vi "HW_Server.vi"(8 "Error In":errorcluster) -> (0 "Error Out":errorcluster)   [LabVIEW 2011]
doc: "This VI will handle communication with Main VI and HW."
uses:
  SubVIs/Controls/TransparencyEffectOperations.ctl
  SubVIs/Controls/Global Stop - Operations.ctl
  SubVIs/Controls/INIT- READ - WRITE.ctl
panel:
  # "HW SERVER"
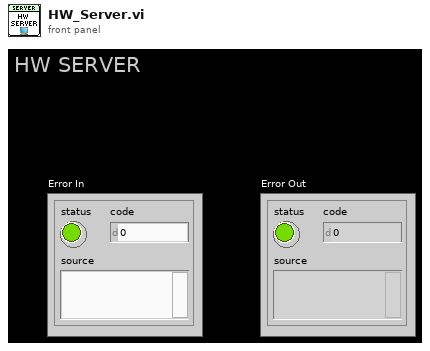
[diagram p1: front panel]
types:
  T1 = typedef "TransparencyEffectOperations.ctl" = enum16{"Show", "Hide 80%", "Hide All"}
  T2 = typedef "Global Stop - Operations.ctl" = enum16{"Stop", "Status", "Init"}
  T3 = typedef "INIT- READ - WRITE.ctl" = enum16{"INIT", "READ", "WRITE"}
  T4 = typedef "HW Server Status.ctl" = enum16{"NO CHASSIS", "NO MODULES", "OK"}
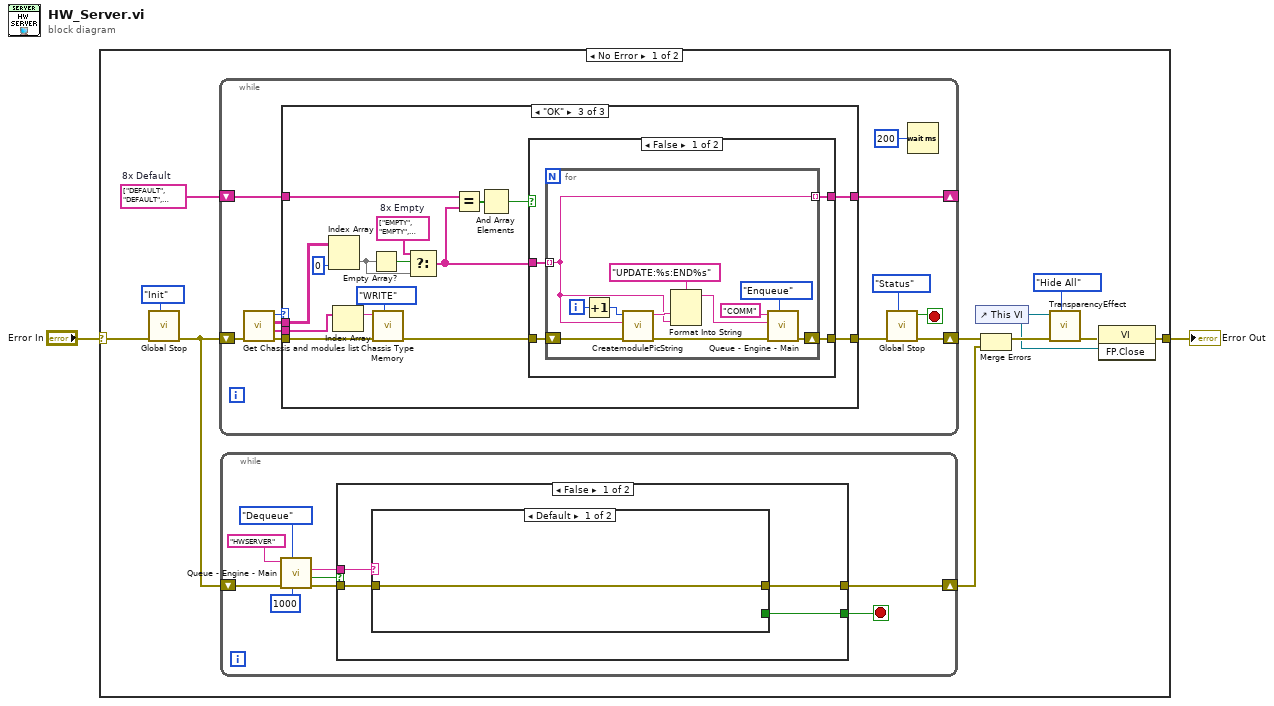
[diagram p0: block diagram]
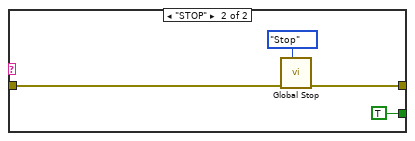
[diagram p2: hidden frame]
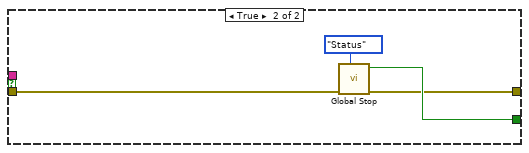
[diagram p3: hidden frame]
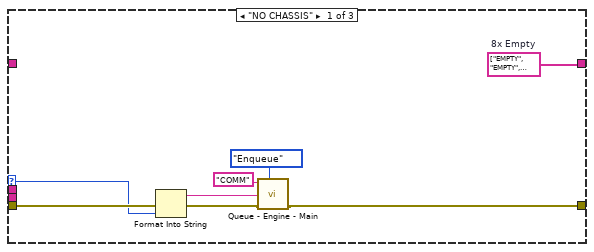
[diagram p4: hidden frame]
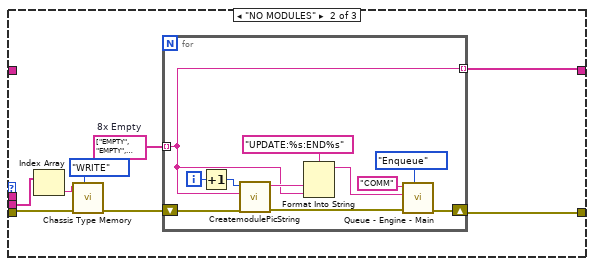
[diagram p5: hidden frame]
diagram:
  n1 = case shown="No Error" "Error In" {
    selector: "Error In" -> [w10 w108]
    tunnel: [w4 w108] -> w2
    frame No Error {
      w13 = string[] ["DEFAULT", "DEFAULT", "DEFAULT", "DEFAULT", "DEFAULT", "DEFAULT", "DEFAULT", "DEFAULT"]  # 8x Default
      n2 = call "Global Stop.vi"("Operation"=Global_Stop_-_Operations."Init", "error in (no error)"=w10) -> ("error out"=w3:errorcluster)  [unwired: 8 in, 1 out]
      n3 = while {
        shift-right: [w40] -> w11
        shift-left: w3 -> [w46]
        shift-right: [w43] -> _
        shift-left: w13 -> [w44]
        stop <- w39 stop-if-true
        n4 = call "Get Chassis and modules list.vi"("error in"=w46) -> ("error out"=w42:errorcluster, "Chassis list"=w36:string[], "Modules Out"=w45:string[][], "Status Out"=w37:T4)  [unwired: 7 in]
        n5 = case shown="\"OK\"" w37 {
          selector: w37 -> [w53 _ _]
          tunnel: w45 -> [_ _ w89]
          tunnel: w44 -> [_ _ w88]
          tunnel: [w55 w61 w81] -> w43
          tunnel: w42 -> [w54 w60 w79]
          tunnel: [w49 w62 w80] -> w41
          tunnel: w36 -> [_ w58 w76]
          frame "NO CHASSIS" {
            w55 = string[] ["EMPTY", "EMPTY", "EMPTY", "EMPTY", "EMPTY", "EMPTY", "EMPTY", "EMPTY"]  # 8x Empty
            n6 = Format Into String(error in=w54, w53) -> (resulting string=w48:string, error out=w50:errorcluster)  [unwired: 2 in]
            n7 = call "Queue - Engine - Main.vi"("Operation"=enum16{"Enqueue", "Dequeue", "Flush", "Release"}."Enqueue", "error in"=w50, "Queue Data In"=w48, "Queue Name In"="COMM") -> ("error out"=w49:errorcluster)  [unwired: 5 in, 2 out]
          }
          frame "NO MODULES" {
            w63 = string[] ["EMPTY", "EMPTY", "EMPTY", "EMPTY", "EMPTY", "EMPTY", "EMPTY", "EMPTY"]  # 8x Empty
            n8 = Index Array(array=w58) -> (element=w57:string)  [unwired: 1 in]
            n9 = call "Chassis Type Memory.vi"("Operation"=INIT-_READ_-_WRITE."WRITE", "Error In"=w60, "Chassis type In"=w57) -> ("Error Out"=w59:errorcluster)  [unwired: 7 in, 1 out]
            n10 = for {
              tunnel: w63 -> [w69] mode=indexing
              shift-right: [w67] -> w62
              shift-left: w59 -> [w70]
              tunnel: [w69] -> w61 mode=indexing
              i -> [w74]
              n11 = Increment(x=w74) -> (x+1=w73:i32)
              n12 = call "CreatemodulePicString.vi"("Error In"=w70, "input string"=w69, "Slot Nr"=w73) -> ("Error Out"=w68:errorcluster, "Pic String Out"=w71:string)  [unwired: 7 in]
              n13 = Format Into String(format string="UPDATE:%s:END%s", w71, w69) -> (resulting string=w66:string)  [unwired: 2 in, 1 out]
              n14 = call "Queue - Engine - Main.vi"("Operation"=enum16{"Enqueue", "Dequeue", "Flush", "Release"}."Enqueue", "error in"=w68, "Queue Data In"=w66, "Queue Name In"="COMM") -> ("error out"=w67:errorcluster)  [unwired: 5 in, 2 out]
            }
          }
          frame "OK" {
            w85 = string[] ["EMPTY", "EMPTY", "EMPTY", "EMPTY", "EMPTY", "EMPTY", "EMPTY", "EMPTY"]  # 8x Empty
            n15 = Index Array(array=w89, index (col)=0 ("disabled index (col)")) -> (element=w83:string[])  [unwired: 1 in]
            n16 = Index Array(array=w76) -> (element=w75:string)  [unwired: 1 in]
            n17 = Empty Array?(array=w83) -> (empty?=w86:bool)
            n18 = call "Chassis Type Memory.vi"("Operation"=INIT-_READ_-_WRITE."WRITE", "Error In"=w79, "Chassis type In"=w75) -> ("Error Out"=w78:errorcluster)  [unwired: 7 in, 1 out]
            n19 = Select(t=w85, s=w86, f=w83) -> (s? t:f=w82:string[])
            n20 = Equal?(x=w88, y=w82) -> (x = y?=w84:bool[])
            n21 = And Array Elements(Boolean array=w84) -> (logical AND=w87:bool)
            n22 = case shown="False" w87 {
              tunnel: w82 -> [w94 w107]
              tunnel: [w93 w106] -> w80
              tunnel: [w92 w107] -> w81
              tunnel: w78 -> [w91 w106]
              frame False {
                n23 = for {
                  tunnel: w94 -> [w100] mode=indexing
                  shift-right: [w96] -> w93
                  shift-left: w91 -> [w101]
                  tunnel: [w100] -> w92 mode=indexing
                  i -> [w105]
                  n24 = Increment(x=w105) -> (x+1=w104:i32)
                  n25 = call "CreatemodulePicString.vi"("Error In"=w101, "input string"=w100, "Slot Nr"=w104) -> ("Error Out"=w97:errorcluster, "Pic String Out"=w102:string)  [unwired: 7 in]
                  n26 = Format Into String(format string="UPDATE:%s:END%s", w102, w100) -> (resulting string=w95:string)  [unwired: 2 in, 1 out]
                  n27 = call "Queue - Engine - Main.vi"("Operation"=enum16{"Enqueue", "Dequeue", "Flush", "Release"}."Enqueue", "error in"=w97, "Queue Data In"=w95, "Queue Name In"="COMM") -> ("error out"=w96:errorcluster)  [unwired: 5 in, 2 out]
                }
              }
              frame True {
              }
            }
          }
        }
        n28 = call "Global Stop.vi"("Operation"=Global_Stop_-_Operations."Status", "error in (no error)"=w41) -> ("error out"=w40:errorcluster, "Stop?"=w39:bool)  [unwired: 8 in]
        n29 = Wait (ms)(milliseconds to wait=u32 200) -> ()  [unwired: 1 out]
      }
      n30 = while {
        shift-right: [w21] -> w12
        shift-left: w3 -> [w19]
        stop <- w22 stop-if-true
        n31 = call "Queue - Engine - Main.vi"("timeout in ms (-1)"=1000, "Operation"=enum16{"Enqueue", "Dequeue", "Flush", "Release"}."Dequeue", "error in"=w19, "Queue Name In"="HWSERVER" ("name")) -> ("error out"=w20:errorcluster, "timed out?"=w14:bool, "Data Out"=w15:string)  [unwired: 5 in]
        n32 = case shown="False" w14 {
          tunnel: w20 -> [w26 w33]
          tunnel: [w25 w32] -> w21
          tunnel: [w24 w34] -> w22
          tunnel: w15 -> [w23 _]
          frame False {
            n33 = case shown="Default" w23 {
              tunnel: w26 -> [w27 w30]
              tunnel: [w27 w29] -> w25
              tunnel: [_ TRUE] -> w24
              frame Default {
              }
              frame "STOP" {
                n34 = call "Global Stop.vi"("Operation"=Global_Stop_-_Operations."Stop", "error in (no error)"=w30) -> ("error out"=w29:errorcluster)  [unwired: 8 in, 1 out]
              }
            }
          }
          frame True {
            n35 = call "Global Stop.vi"("Operation"=Global_Stop_-_Operations."Status", "error in (no error)"=w33) -> ("error out"=w32:errorcluster, "Stop?"=w34:bool)  [unwired: 8 in]
          }
        }
      }
      n36 = control-ref of="This VI"() -> (w6:refnum<vi>)
      n37 = Merge Errors(w11, w12) -> (w7:errorcluster)
      n38 = call "TransparencyEffect.vi"("Operation"=TransparencyEffectOperations."Hide All", "error in"=w7, "VI Ref in"=w6) -> ("error out"=w5:errorcluster)  [unwired: 8 in]
      n39 = invoke class="VI" method="FP.Close"(reference=w6, error in=w5) -> (error out=w4:errorcluster)  [unwired: 1 in, 2 out]
    }
    frame Error {
    }
  }
  "Error Out" <- w2
